vi "RW_Redis.vi"(8 "error in":errorcluster, 10 "command":string="PING", 11 "TCP session in":refnum<k5>) -> (0 "error out":errorcluster, 2 "Data":T1, 3 "TCP session out":refnum<k5>)   [LabVIEW 2023]
uses:
  Controls/redis-data.ctl
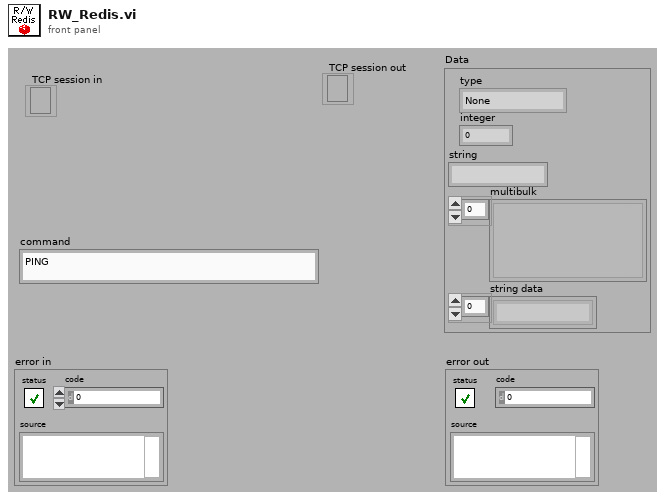
[diagram p1: front panel]
types:
  T1 = typedef "redis-data.ctl" = cluster{"type":enum16{"None", "Error", "Status", "Nil", "Integer", "String", "Multibulk"}, "integer":i64, "string":string, "multibulk":variant[], "string data":string[]}
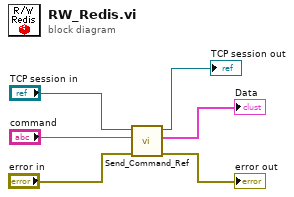
[diagram p0: block diagram]
diagram:
  n1 = call "Send_Command_Ref.vi"("error in"="error in", "command"="command", "TCP session in"="TCP session in") -> ("error out"=→"error out":errorcluster, "Data"=→"Data":T1, "TCP session out"=→"TCP session out":refnum<k5>)  [unwired: 6 in]
